vi "ClickedPosition.vi"(9 "Number of Columns":u32=8, 10 "Number of Rows":u32, 11 "Input Array":dbl[][](array[numeric])) -> (2 "Clicked index":i32[](array[numeric]))   [LabVIEW 2019]
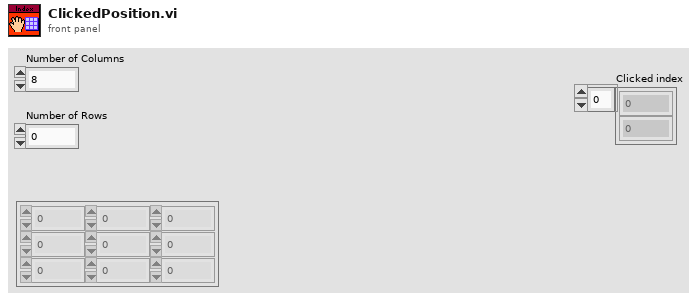
[diagram p1: front panel]
types:
  T1 = typedef "LVPoint32TypeDef.ctl" = cluster{"Horizontal":i32, "Vertical":i32}
  T2 = typedef "LVPositionTypeDef.ctl" = cluster{"Left":i32, "Top":i32}
  T3 = typedef "LVBoundsTypeDef.ctl" = cluster{"Width":u32, "Height":u32}
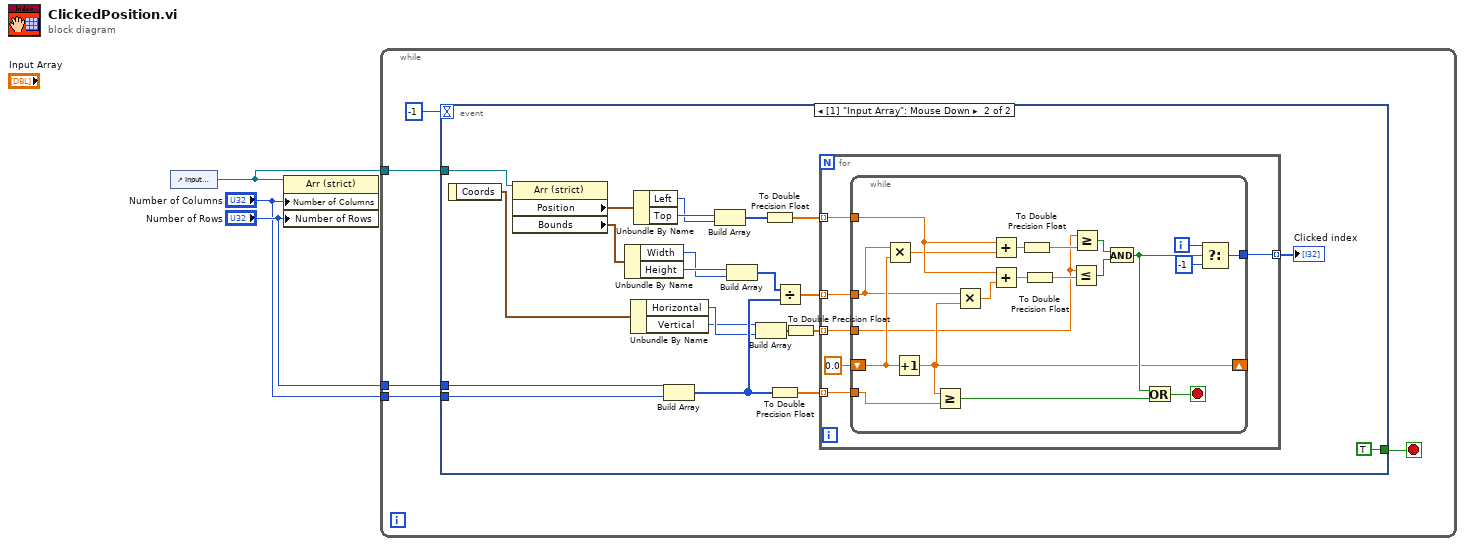
[diagram p0: block diagram]
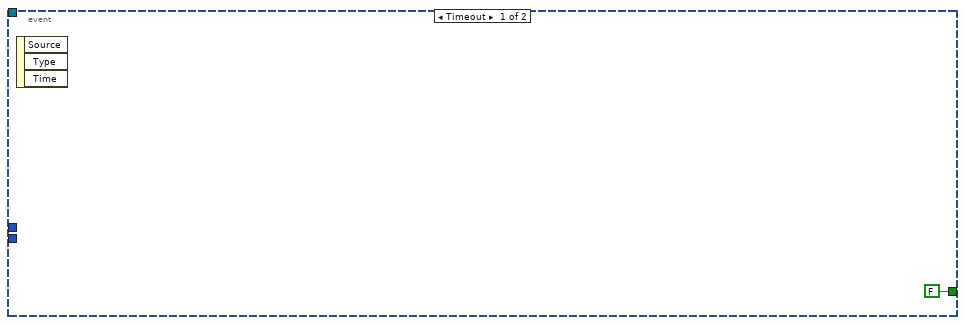
[diagram p2: hidden frame]
diagram:
  n1 = control-ref of="Input Array"() -> (w1:refnum<vi>)
  n2 = property on="Property Node" class="Arr (strict)"(reference=w1, "Number of Columns"="Number of Columns", "Number of Rows"="Number of Rows") -> ()  [unwired: 1 in, 2 out]
  n3 = while {
    tunnel: "Number of Columns" -> [w7]
    tunnel: "Number of Rows" -> [w5]
    tunnel: w1 -> [w4]
    stop <- w6 stop-if-true
    n4 = event shown="[1] \"Input Array\": Mouse Down" {
      selector: _ -> [_ _]
      dyn-events: _ -> [_ _]
      timeout: -1 -> [_ _]
      tunnel: w7 -> [_ w13]
      tunnel: [FALSE ("Exit") TRUE ("Exit")] -> w6
      tunnel: w5 -> [_ w14]
      tunnel: w4 -> [_ w12]
      event Timeout {
        n5 = event-data() -> ()  [unwired: 1 in, 3 out]
      }
      event "Input Array": Mouse Down {
        n6 = event-data() -> ("Coords"=w29:T1)  [unwired: 1 in]
        n7 = property on="Property Node" class="Arr (strict)"(reference=w12) -> ("Position"=w31:T2, "Bounds"=w30:T3)  [unwired: 1 in, 2 out]
        n8 = Unbundle By Name(w30) -> ("Width"=w25:u32, "Height"=w26:u32)
        n9 = Unbundle By Name(w29) -> ("Horizontal"=w19:i32, "Vertical"=w18:i32)
        n10 = Unbundle By Name(w31) -> ("Left"=w27:i32, "Top"=w28:i32)
        n11 = Build Array(w14, w13) -> (w22:u32[])
        n12 = Build Array(w28, w27) -> (w24:i32[])
        n13 = Build Array(w26, w25) -> (w23:u32[])
        n14 = Build Array(w18, w19) -> (w20:i32[])
        n15 = To Double Precision Float(number=w24) -> (double precision float=w17:dbl[])
        n16 = To Double Precision Float(number=w22) -> (double precision float=w16:dbl[])
        n17 = Divide(x=w23, y=w22) -> (x/y=w21:dbl[])
        n18 = To Double Precision Float(number=w20) -> (double precision float=w15:dbl[])
        n19 = for {
          tunnel: w17 -> [w33] mode=indexing
          tunnel: w16 -> [w37] mode=indexing
          tunnel: w21 -> [w34] mode=indexing
          tunnel: w15 -> [w35] mode=indexing
          tunnel: [w32] -> w11 mode=indexing
          n20 = while {
            tunnel: w37 -> [w57]
            tunnel: w35 -> [w38]
            tunnel: w34 -> [w39]
            tunnel: w33 -> [w44]
            tunnel: [w46] -> w32
            shift-right: [w43] -> _
            shift-left: 0.0 -> [w42]
            i -> [w47]
            stop <- w55 stop-if-true
            n21 = Multiply(x=w39, y=w42) -> (x*y=w41:dbl)
            n22 = Increment(x=w42) -> (x+1=w43:dbl)
            n23 = Greater Or Equal?(x=w43, y=w57) -> (x >= y?=w56:bool)
            n24 = Multiply(x=w39, y=w43) -> (x*y=w40:dbl)
            n25 = Add(x=w44, y=w41) -> (x+y=w52:dbl)
            n26 = Add(x=w44, y=w40) -> (x+y=w54:dbl)
            n27 = To Double Precision Float(number=w52) -> (double precision float=w51:dbl)
            n28 = To Double Precision Float(number=w54) -> (double precision float=w53:dbl)
            n29 = Less Or Equal?(x=w38, y=w53) -> (x <= y?=w49:bool)
            n30 = Greater Or Equal?(x=w38, y=w51) -> (x >= y?=w50:bool)
            n31 = And(x=w50, y=w49) -> (x .and. y?=w45:bool)
            n32 = Or(x=w45, y=w56) -> (x .or. y?=w55:bool)
            n33 = Select(t=w47, s=w45, f=-1) -> (s? t:f=w46:i32)
          }
        }
        "Clicked index" <- w11
      }
    }
  }
